vi "Confidence Interval (Polynomial).vi"(0 "Y":dbl[](array[numeric]), 1 "confidence level":dbl=0.95 format="%.2f", 5 "X":dbl[](array[numeric]), 7 "Weight":dbl[](array[numeric]), 9 "Polynomial Coefficients":dbl[](array[numeric])) -> (4 "Upper Bound":dbl[](array[numeric]), 6 "Lower Bound":dbl[](array[numeric]), 8 "Delta Polynomial Coefficients":dbl[](array[numeric]), 15 "error":i32)   [LabVIEW 2020, in "NI_AALPro.lvlib"]
doc: "Calculates statistical intervals of the best polynomial fit for a data set (<B>X</B>, <B>Y</B>)."
uses:
  NI_AALPro.lvlib
  <resource>/lvanlys.dll
panel:
  out "Lower Coefficients":dbl[](array[numeric])
  out "Upper Coefficients":dbl[](array[numeric])
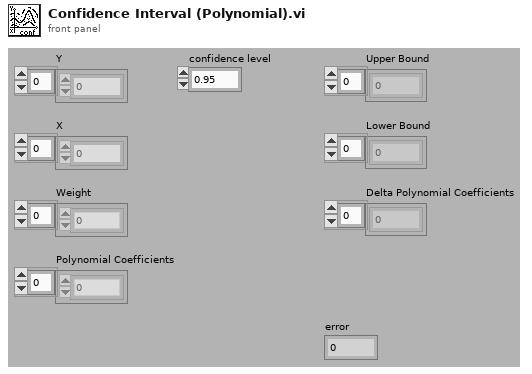
[diagram p1: front panel]
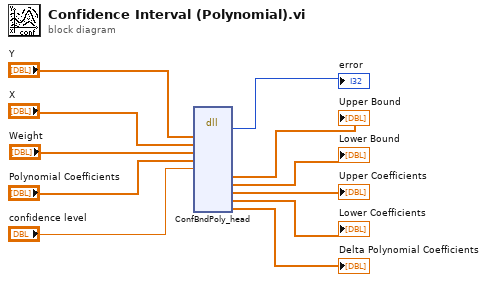
[diagram p0: block diagram]
diagram:
  n1 = dll-call lib="C:/Program Files (x86)/National Instruments/LabVIEW 2020/resource/lvanlys.*" fn="ConfBndPoly_head"("y"="Y", "x"="X", "weight"="Weight", "polyCoef"="Polynomial Coefficients", "confidentLevel"="confidence level") -> ("return type"=→"error":i32, "upper"=→"Upper Bound":dbl[], "lower"=→"Lower Bound":dbl[], "upperCoef"=→"Upper Coefficients":dbl[], "lowerCoef"=→"Lower Coefficients":dbl[], "deltaCoef"=→"Delta Polynomial Coefficients":dbl[])  [unwired: 8 in, 7 out]
